vi "STAGE+mono+counter_edit26.vi"() -> ()   [LabVIEW 2017]
panel:
  out "Timeout":bool
  out "PROGRESS":u8(slide) max=10 step=10 scale=0.0..1.0
  in  "?":enum32{"Scan Data", "Scans", "RT Data"}(tab)
  out "Spectrum":cluster{dbl[], dbl[]}(graph)
  out "Decay":cluster{dbl[], dbl[]}[](graph)
  in  "Collect Data!":bool
  out "Waveform Graph":waveform(dbl)[](graph)
  out "?":i32(knob) scale=0.0..1000000.0
  out "Photon Counts":dbl
  in  "Wavelength":dbl
  in  "Show Real Time Data":bool
  in  "?":enum32{"DELAY", "COUNTER", "MONO", "PLOT"}(tab)
  in  "Data File Path":path
  out "Final time [ps]":dbl
  out "Current time [ps]":dbl
  out "Initial time [ps]":dbl
  in  "Set this as t0":bool
  in  "Axis":i32=1
  in  "Motor ON":bool
  in  "Motor OFF":bool
  out "Current Position [mm]":dbl
  out "Final Position [mm]":dbl
  in  "Data Points":i32=100
  out "Current Point":i32
  in  "Step Size [um]":i32=10
  in  "Target [mm]":dbl format="%.3f"
  in  "Move":bool
  out "Initial position [mm]":dbl
  in  "GPIB address":string="23"
  in  "Count Mode":u16(ring) items=["A,B for Preset T", "A-B for Preset T", "A+B for Preset T", "A for Preset B"]
  in  "Trigger mode":u16(ring) items=["10 MHz"=0, "Input 2"=2, "Input T"=3]
  in  "Channel A Input":u16(ring)=1 items=["10 MHz", "Input 1"]
  in  "Channel B Input":u16(ring)=2 items=["Input 1"=1, "Input 2"=2]
  in  "Number of Measurements\n to take at one point/ Number of Periods":u16=1 min=1 max=2000 step=1
  in  "Time between measurements\n at one point (s)/Dwell Time":dbl=0.002 min=0.002 max=60.0 step=0.001
  in  "gate mode (CW:0)":i16(slide) scale=0.0..2.0 scale format="%.2f"
  out "Counts":i32
  in  "Integrating time \nin 10^-7 sec":dbl=10000000.0
  in  "Discriminator Level (mV)":dbl min=-300.0 max=300.0 step=0.2
  in  "Discriminator Slope":bool
  in  "Channel":i16 min=0 max=2 step=1
  out "Grating #":dbl
  out "Blaze angle":dbl
  out "Grooves/mm":dbl
  out "Mono port":T1(ring)
  out "Time delay":u32=450000 min=1
  in  "Step size":dbl=10.0 min=0.0
  in  "Scan to":i32=4000
  in  "Scan from":i32=2600
  out "Current wavelength":dbl
  in  "?":bool
  in  "NEW UNIT":T2(ring)
  in  "Array":dbl[](array[numeric])
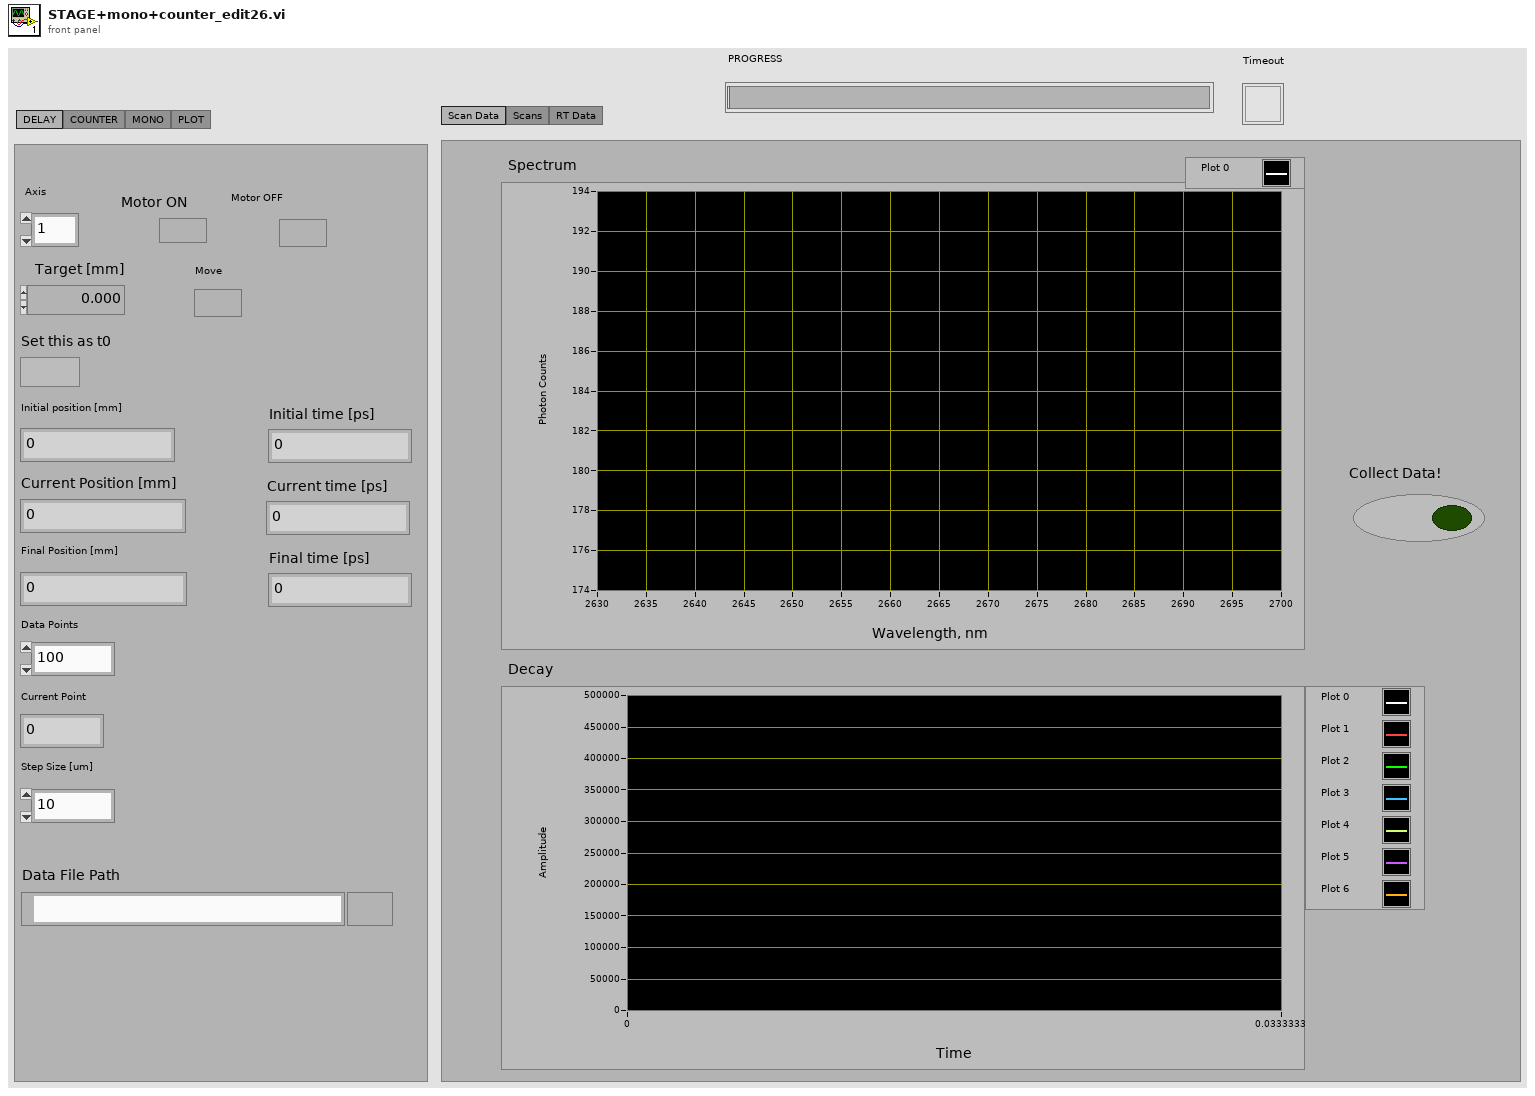
[diagram p1: front panel]
types:
  T1 = enum8{"COM 1", "COM 2", "COM 3", "COM 4", "COM 5", "COM 6", "COM 7", "COM 8", "COM 9"}
  T2 = enum16{"centi-Microns", " Nanometers", "   Angstroms"}
  T3 = cluster{"input XON/XOFF":bool, "input HW Handshake":bool, "input alt HW HShk":bool, "output XON/XOFF":bool, "output HW Handshake":bool, "output alt HW HShk":bool, "XOFF byte":u8, "XON byte":u8, "parity error byte":u16}
  T4 = enum16{"no parity", "odd parity", "even parity", "mark parity", "space parity"}
  T5 = enum16{"open", "replace", "create", "open or create", "replace or create", "replace or create with confirmation"}
  T6 = typedef "NI_Matrix.lvlib/RealMatrix.ctl" = dbl[][]
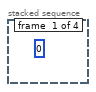
[diagram p2: hidden frame]
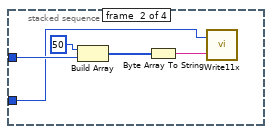
[diagram p3: hidden frame]
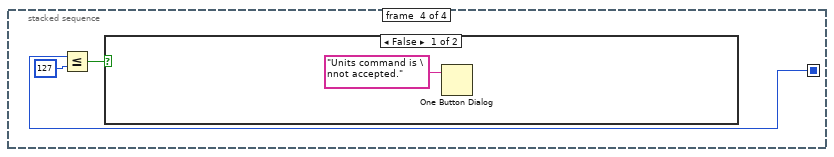
[diagram p4: hidden frame]
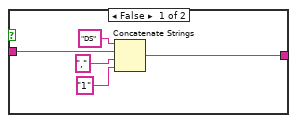
[diagram p7: hidden frame]
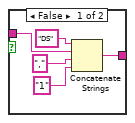
[diagram p9: hidden frame]
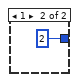
[diagram p13: hidden frame]
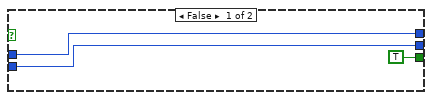
[diagram p14: hidden frame]
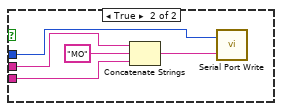
[diagram p15: hidden frame]
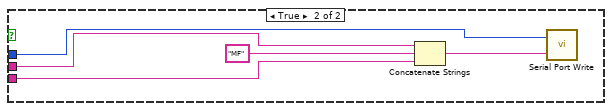
[diagram p16: hidden frame]
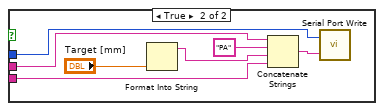
[diagram p17: hidden frame]
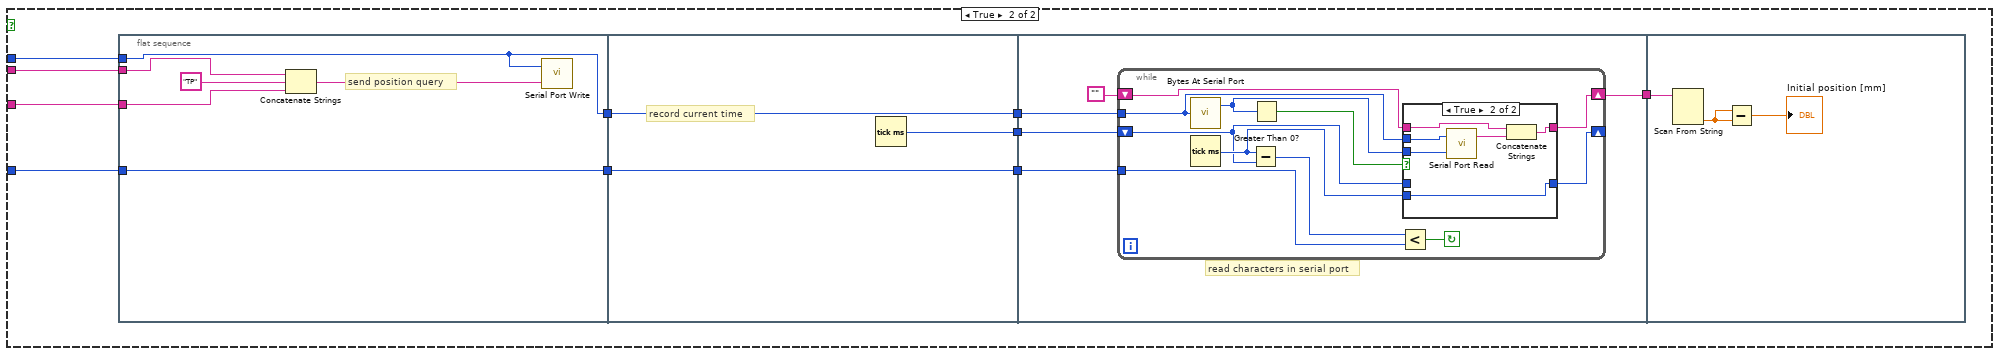
[diagram p18: hidden frame]
diagram:
  w35 = u32 19200  # baud rate
  w34 = u16 8  # data bits
  w33 = enum16{"1 bit", "1.5 bits", "2 bits"}."1 bit"  # stop bits
  w37 = T4."no parity"  # parity
  w17 = 4  # 0=COM1 so n=COM(n+1)
  w36 = u16 1024  # buffer size
  n1 = flat-sequence {
    tunnel: [w40] -> w9
    tunnel: [w39] -> w10
    frame #0 {
      n2 = call "CM Com Read ini.vi"() -> ("Mono port"=w39:T1, "time delay1"=w40:u32)  [unwired: 7 in]
    }
  }
  n3 = stacked-sequence {
    seq-local: [_ _ w48 _] -> [_ _ _ w55]
    tunnel: "NEW UNIT" -> [_ w42 _ _]
    tunnel: w9 -> [_ w41 w46 _]
    tunnel: w10 -> [_ _ w47 _]
    frame #0 {
      (unwired) u8 0
    }
    frame #1 {
      n4 = Build Array(u8 50, w42) -> (w44:u16[])
      n5 = Byte Array To String(unsigned byte array=w44) -> (string=w43:string)
      n6 = call "Write11x.vi"("string to write"=w43, "port number"=w41) -> ()  [unwired: 1 out]
    }
    frame #2 {
      n7 = call "Read11x.vi"("response size"=2, "timeout count"=w47, "port number"=w46) -> ("rcv index"=w49:u8[])  [unwired: 2 out]
      n8 = Index Array(array=w49, index=1) -> ()  [unwired: 1 out]
      n9 = Index Array(array=w49, index=0) -> (element=w48:u8)
    }
    frame #3 {
      n10 = Less Or Equal?(x=w55, y=127) -> (x <= y?=w53:bool)
      n11 = case shown="False" w53 {
        frame False {
          n12 = One Button Dialog(message="Units command is \nnot accepted.") -> ()  [unwired: 1 in, 1 out]
        }
        frame True {
        }
      }
    }
  }
  n13 = call "CM Serial Port Setup.vi"("COM port"=w10, "time delay"=w9) -> ("time delay1"=w1:u32, "DK port Out"=w2:T1, "error code"=w28:i32)  [unwired: 7 in]
  n14 = Equal To 0?(x=w28) -> (x = 0?=w27:bool)
  n15 = case shown="True" w27 {
    tunnel: w2 -> [w59 w62]
    tunnel: w1 -> [w58 w61]
    tunnel: [w59 w62] -> w14
    tunnel: [w58 w61] -> w13
    tunnel: [TRUE FALSE] -> w12
    frame False {
    }
    frame True {
      n16 = call "CM Com Write ini.vi"("time delay1"=w62, "Mono port"=w61) -> ()  [unwired: 7 in]
      n17 = local write "Mono port"(w62) -> ()
      n18 = local write "Time delay"(w61) -> ()
    }
  }
  n19 = call "Query11x.vi"("port number"=w2, "QUERY"=u16 4, "time delay"=w1) -> ("STATUS MESSAGE"=→"Grating #":u16)  [unwired: 3 out]
  n20 = call "Query11x.vi"("port number"=w2, "QUERY"=u16 2, "time delay"=w1) -> ("STATUS MESSAGE"=→"Grooves/mm":u16)  [unwired: 3 out]
  n21 = call "Query11x.vi"("port number"=w2, "QUERY"=u16 3, "time delay"=w1) -> ("STATUS MESSAGE"=→"Blaze angle":u16)  [unwired: 3 out]
  n22 = call <vilib>:"Serial Port Init.vi"("flow control etc."=T3 {"input XON/XOFF"=FALSE, "input HW Handshake"=FALSE, "input alt HW HShk"=FALSE, "output XON/XOFF"=FALSE, "output HW Handshake"=FALSE, "output alt HW HShk"=FALSE, "XOFF byte"=13, "XON byte"=11, "parity error byte"=0}, "parity"=w37, "buffer size"=w36, "stop bits"=w33, "data bits"=w34, "baud rate"=w35, "port number"=w17) -> ("error code"=w32:i32)
  n23 = Concatenate Strings("\r", "\n") -> (w29:string)
  n24 = while {
    tunnel: w13 -> [w65]
    tunnel: w14 -> [w64]
    stop <- TRUE continue-if-true
    n25 = case shown="True" "?" {
      tunnel: w65 -> [_ w68]
      tunnel: w64 -> [_ w67]
      frame False {
      }
      frame True {
        n26 = Two Button Dialog(message="Do you want to change grating?", 1:"No" ("F button name (\"Cancel\")"), 2:"Yes" ("T button name (\"OK\")")) -> (T button?=w69:bool)
        n27 = case shown="True" w69 {
          tunnel: w68 -> [_ w74]
          tunnel: w67 -> [_ w73]
          frame False {
          }
          frame True {
            n28 = Two Button Dialog(message="Disable voltage from PMT", 1:"Do not swich grating" ("F button name (\"Cancel\")"), 2:"Done" ("T button name (\"OK\")")) -> (T button?=w75:bool)
            n29 = case shown="True" w75 {
              tunnel: w74 -> [_ w87]
              tunnel: w73 -> [_ w86]
              frame False {
              }
              frame True {
                n30 = flat-sequence {
                  tunnel: w87 -> [w91]
                  tunnel: [w91] -> w81
                  tunnel: w86 -> [w90]
                  tunnel: [w90] -> w80
                  tunnel: [w88] -> w79
                  tunnel: w81 -> [w96]
                  tunnel: [w96] -> w84
                  tunnel: w80 -> [w97]
                  tunnel: [w97] -> w83
                  tunnel: w79 -> [w95]
                  tunnel: [w95] -> w82
                  tunnel: w84 -> [w101]
                  tunnel: w83 -> [w102]
                  tunnel: [w100] -> w85
                  tunnel: w82 -> [w100]
                  frame #0 {
                    n31 = local read "Grating #"() -> (w89:dbl)
                    n32 = case shown="2, Default" w89 {
                      tunnel: [1 2] -> w88
                      frame 2, Default {
                      }
                      frame 1 {
                      }
                    }
                    n33 = call "Select11x2.vi"("time delay"=w91, "NEW GRT?"=w88, "port number"=w90) -> ()  [unwired: 3 out]
                  }
                  frame #1 {
                    n34 = call "Query11x.vi"("port number"=w97, "QUERY"=u16 2, "time delay"=w96) -> ("STATUS MESSAGE"=w94:u16)  [unwired: 3 out]
                    n35 = local write "Grooves/mm"(w94) -> ()
                  }
                  frame #2 {
                    n36 = Divide(x=w101, y=i16 100 ("device (1)")) -> (x/y=w103:dbl)
                    n37 = call "Query11x.vi"("port number"=w102, "QUERY"=u16 3, "time delay"=w103) -> ("STATUS MESSAGE"=w99:u16)  [unwired: 3 out]
                    n38 = local write "Blaze angle"(w99) -> ()
                  }
                }
                n39 = local write "Grating #"(w85) -> ()
              }
            }
          }
        }
      }
    }
  }
  n40 = while {
    tunnel: w17 -> [w120]
    tunnel: w29 -> [w121]
    tunnel: w32 -> [_]
    tunnel: "Axis" -> [w118]
    stop <- TRUE continue-if-true
    w119 = u32 200  # timeout
    n41 = Format Into String(w118) -> (resulting string=w122:string)  [unwired: 3 in, 1 out]
    n42 = flat-sequence {
      tunnel: w122 -> [w127]
      tunnel: w121 -> [w126]
      tunnel: w120 -> [w128]
      tunnel: w119 -> [w125]
      tunnel: [w127] -> w117
      tunnel: [w126] -> w116
      tunnel: [w128] -> w115
      tunnel: [w125] -> w114
      tunnel: w117 -> [w138]
      tunnel: w116 -> [w137]
      tunnel: w115 -> [w139]
      tunnel: w114 -> [w135]
      tunnel: [w138] -> w113
      tunnel: [w137] -> w112
      tunnel: [w139] -> w111
      tunnel: [w135] -> w110
      tunnel: w113 -> [w148]
      tunnel: w112 -> [w147]
      tunnel: w111 -> [w149]
      tunnel: w110 -> [w145]
      tunnel: [w148] -> w109
      tunnel: [w147] -> w108
      tunnel: [w149] -> w107
      tunnel: [w145] -> w106
      tunnel: w109 -> [w161]
      tunnel: w108 -> [w158]
      tunnel: w107 -> [w160]
      tunnel: w106 -> [w159]
      frame #0 {
        n43 = case shown="False" "Motor ON" {
          tunnel: w128 -> [_ w134]
          tunnel: w127 -> [_ w131]
          tunnel: w126 -> [_ w130]
          frame False {
          }
          frame True {
            n44 = Concatenate Strings(w131, "MO" ("Substring"), w130) -> (w132:string)
            n45 = call <vilib>:"Serial Port Write.vi"("string to write"=w132, "port number"=w134) -> ()  [unwired: 1 out]
          }
        }
      }
      frame #1 {
        n46 = case shown="False" "Motor OFF" {
          tunnel: w139 -> [_ w144]
          tunnel: w138 -> [_ w141]
          tunnel: w137 -> [_ w140]
          frame False {
          }
          frame True {
            n47 = Concatenate Strings(w141, "MF" ("Substring"), w140) -> (w142:string)
            n48 = call <vilib>:"Serial Port Write.vi"("string to write"=w142, "port number"=w144) -> ()  [unwired: 1 out]
          }
        }
      }
      frame #2 {
        n49 = case shown="False" "Move" {
          tunnel: w149 -> [_ w156]
          tunnel: w148 -> [_ w153]
          tunnel: w147 -> [_ w152]
          frame False {
          }
          frame True {
            n50 = Format Into String("Target [mm]") -> (resulting string=w150:string)  [unwired: 3 in, 1 out]
            n51 = Concatenate Strings(w153, "PA" ("Substring"), w150, w152) -> (w154:string)
            n52 = call <vilib>:"Serial Port Write.vi"("string to write"=w154, "port number"=w156) -> ()  [unwired: 1 out]
          }
        }
      }
      frame #3 {
        n53 = case shown="False" "Set this as t0" {
          tunnel: w161 -> [_ w171]
          tunnel: w160 -> [_ w170]
          tunnel: w159 -> [_ w169]
          tunnel: w158 -> [_ w168]
          frame False {
          }
          frame True {
            n54 = flat-sequence {
              tunnel: w171 -> [w175]
              tunnel: w170 -> [w174]
              tunnel: [w174] -> w167
              tunnel: w169 -> [w172]
              tunnel: [w172] -> w166
              tunnel: w168 -> [w173]
              tunnel: w167 -> [w179]
              tunnel: [w179] -> w165
              tunnel: w166 -> [w178]
              tunnel: [w178] -> w164
              tunnel: [w180] -> w163
              tunnel: w165 -> [w185]
              tunnel: w164 -> [w183]
              tunnel: w163 -> [w182]
              tunnel: [w181] -> w162
              tunnel: w162 -> [w207]
              frame #0 {
                # "send position query"
                n55 = Concatenate Strings(w175, "TP" ("Substring"), w173) -> (w176:string)
                n56 = call <vilib>:"Serial Port Write.vi"("string to write"=w176, "port number"=w174) -> ()  [unwired: 1 out]
              }
              frame #1 {
                # "record current time"
                n57 = Tick Count (ms)() -> (millisecond timer value=w180:u32)
              }
              frame #2 {
                # "read characters in serial port"
                n58 = while {
                  shift-left: w182 -> [w186]
                  shift-right: [w187] -> _
                  tunnel: w183 -> [w190]
                  shift-left: "" -> [w193]
                  shift-right: [w192] -> w181
                  tunnel: w185 -> [w194]
                  stop <- w189 continue-if-true
                  n59 = call <vilib>:"Bytes At Serial Port.vi"("port number"=w194) -> ("byte count"=w195:u32)  [unwired: 1 out]
                  n60 = Tick Count (ms)() -> (millisecond timer value=w188:u32)
                  n61 = Subtract(x=w188, y=w186) -> (x-y=w191:u32)
                  n62 = Greater Than 0?(x=w195) -> (x > 0?=w196:bool)
                  n63 = Less?(x=w191, y=w190) -> (x < y?=w189:bool)
                  n64 = case shown="True" w196 {
                    tunnel: w195 -> [_ w204]
                    tunnel: w194 -> [_ w203]
                    tunnel: w193 -> [w198 w201]
                    tunnel: [w198 w200] -> w192
                    tunnel: [w197 w199] -> w187
                    tunnel: w188 -> [_ w199]
                    tunnel: w186 -> [w197 _]
                    frame False {
                    }
                    frame True {
                      n65 = call <vilib>:"Serial Port Read.vi"("requested byte count"=w204, "port number"=w203) -> ("string read"=w202:string)  [unwired: 1 out]
                      n66 = Concatenate Strings(w201, w202) -> (w200:string)
                    }
                  }
                }
              }
              frame #3 {
                n67 = Scan From String(input string=w207) -> (output 1=w205:dbl)  [unwired: 4 in, 3 out]
                n68 = Subtract(x=w205, y=w205) -> (x-y=→"Initial position [mm]":dbl)
              }
            }
          }
        }
      }
    }
    n69 = Wait Until Next ms Multiple(millisecond multiple=u32 50) -> ()  [unwired: 1 out]
  }
  n70 = while {
    tunnel: "GPIB address" -> [w211]
    tunnel: w14 -> [w210]
    tunnel: w13 -> [w209]
    tunnel: w12 -> [w208]
    stop <- TRUE continue-if-true
    n71 = case shown="True" "Show Real Time Data" {
      tunnel: w211 -> [_ w220]
      tunnel: w210 -> [_ w217]
      tunnel: w209 -> [_ w214]
      tunnel: w208 -> [_ w219]
      frame False {
      }
      frame True {
        n72 = flat-sequence {
          tunnel: w220 -> [w249]
          tunnel: "Wavelength" -> [w250]
          tunnel: [w250] -> w231
          tunnel: [w239] -> w230
          tunnel: [w240] -> w229
          tunnel: [w249] -> w228
          tunnel: w214 -> [w240]
          tunnel: w217 -> [w239]
          tunnel: w219 -> [_]
          tunnel: [w238] -> w215
          tunnel: w214 -> [w238]
          tunnel: [w258] -> w227
          tunnel: [w257] -> w226
          tunnel: [w255] -> w225
          tunnel: w231 -> [w253]
          tunnel: w230 -> [w258]
          tunnel: w229 -> [w257]
          tunnel: w228 -> [w255]
          tunnel: [w251] -> w216
          tunnel: w215 -> [w251]
          tunnel: w227 -> [_]
          tunnel: w226 -> [_]
          tunnel: w225 -> [w261]
          tunnel: [w261] -> w224
          tunnel: w217 -> [w260]
          tunnel: w216 -> [w259]
          tunnel: w224 -> [w270]
          tunnel: [w270] -> w223
          tunnel: w223 -> [w320]
          tunnel: [w320] -> w222
          tunnel: w222 -> [w321]
          tunnel: [w321] -> w221
          tunnel: w221 -> [w331]
          frame #0 {
            n73 = call "Query11x.vi"("port number"=w239, "QUERY"=u16 0, "time delay"=w240) -> ("timeout"=w236:bool, "STATUS MESSAGE"=w235:u16)  [unwired: 2 out]
            n74 = call "Query11x.vi"("port number"=w239, "QUERY"=u16 2, "time delay"=w240) -> ("timeout"=w247:bool, "STATUS MESSAGE"=w246:u16)  [unwired: 2 out]
            n75 = call "Query11x.vi"("port number"=w239, "QUERY"=u16 4, "time delay"=w240) -> ("timeout"=w241:bool, "STATUS MESSAGE"=w242:u16)  [unwired: 2 out]
            n76 = call "Query11x.vi"("port number"=w239, "QUERY"=u16 3, "time delay"=w240) -> ("timeout"=→"Timeout":bool, "STATUS MESSAGE"=w244:u16)  [unwired: 2 out]
            n77 = local write "Timeout"(w236) -> ()
            n78 = local write "Timeout"(w247) -> ()
            n79 = local write "Grooves/mm"(w246) -> ()
            n80 = local write "Timeout"(w241) -> ()
            n81 = local write "Grating #"(w242) -> ()
            n82 = Divide(x=w235, y=10 ("Numeric")) -> (x/y=w233:dbl)
            n83 = local write "Current wavelength"(w233) -> ()
            n84 = local write "Blaze angle"(w244) -> ()
          }
          frame #1 {
            n85 = Multiply(x=w253, y=1) -> (x*y=w252:dbl)
            n86 = call "Goto11x.vi"("time delay"=w257, "WAVELENGTH"=w252, "port number"=w258) -> ("timeout"=w256:bool)  [unwired: 2 out]
            n87 = local write "Timeout"(w256) -> ()
          }
          frame #2 {
            # "set counter time in 10^-7 seconds in CW"
            n88 = call "Query11x.vi"("port number"=w260, "QUERY"=0, "time delay"=w259) -> ("timeout"=w265:bool, "STATUS MESSAGE"=w264:u16)  [unwired: 2 out]
            n89 = local write "Timeout"(w265) -> ()
            n90 = Divide(x=w264, y=1) -> (x/y=w263:dbl)
            n91 = local write "Current wavelength"(w263) -> ()
          }
          frame #3 {
            # "Configures discriminator."
            n92 = flat-sequence {
              tunnel: w270 -> [w277]
              tunnel: [w277] -> w276
              tunnel: [w284] -> w275
              tunnel: [w282] -> w274
              tunnel: w269 -> [w283]
              tunnel: w276 -> [w282]
              tunnel: w271 -> [w281]
              tunnel: w275 -> [w303]
              tunnel: [w304] -> w273
              tunnel: w274 -> [w302]
              tunnel: [w302] -> w272
              tunnel: w271 -> [w300]
              tunnel: w273 -> [w316]
              tunnel: w272 -> [w315]
              tunnel: w267 -> [w310]
              tunnel: w271 -> [w309]
              frame #0 {
                # "Flush I/O buffers."
                n93 = for {
                  N: 5 -> [_]
                  tunnel: w277 -> [w279]
                  n94 = GPIB Write(0:w279, 1:"\r") -> ()  [unwired: 3 in, 2 out]
                }
              }
              frame #1 {
                # "Set discriminator slope."
                n95 = case shown="True" w283 {
                  tunnel: [w290 w295] -> w285
                  tunnel: w281 -> [w289 w294]
                  frame False {
                    n96 = Concatenate Strings("DS", w289, ",", "1") -> (w290:string)
                  }
                  frame True {
                    n97 = Concatenate Strings("DS", w294, ",", "0") -> (w295:string)
                  }
                }
                n98 = GPIB Write(0:w282, 1:w285, 2:5) -> (6:w284:errorcluster)  [unwired: 2 in, 1 out]
              }
              frame #2 {
                # "Set discriminator mode to fixed."
                n99 = Concatenate Strings("DM", w300, ",", "0") -> (w299:string)
                n100 = GPIB Write(0:w302, 1:w299, 2:5, 3:w303) -> (6:w304:errorcluster)  [unwired: 1 in, 1 out]
              }
              frame #3 {
                # "Set discriminator level.\nMust be between +300 and -300 mV."
                n101 = Divide(x=w310, y=1000.0) -> (x/y=w318:dbl)
                n102 = Number To Fractional String(number=w318, precision (6)=i16 4) -> (F-format string=w307:string)  [unwired: 2 in]
                n103 = Concatenate Strings("DL", w309, ",", w307) -> (w314:string)
                n104 = GPIB Write(0:w315, 1:w314, 2:5, 3:w316) -> (6:w311:errorcluster)  [unwired: 1 in, 1 out]
                n105 = call <vilib>:"General Error Handler.vi"("type of dialog (OK msg:1)"=1, "error in (no error)"=w311) -> ()  [unwired: 9 in, 5 out]
              }
            }
            n106 = local read "Discriminator Slope"() -> (w269:bool)
            n107 = local read "Channel"() -> (w268:i16)
            n108 = Number To Decimal String(number=w268) -> (decimal integer string=w271:string)  [unwired: 1 in]
            n109 = local read "Discriminator Level (mV)"() -> (w267:dbl)
          }
          frame #4 {
            n110 = call "Start.vi"("GPIB Address"=w320) -> ()  [unwired: 9 in]
          }
          frame #5 {
            # "Wait for Scan to Finish"
            n111 = for {
              N: 1 -> [_]
              tunnel: w321 -> [w323]
              n112 = while {
                tunnel: w323 -> [w324]
                stop <- w326 stop-if-true
                n113 = call "ScanDone.vi"("Wait (ms)"=1000, "GPIB Address"=w324) -> ("Scan Finished?"=w326:bool)
              }
            }
          }
          frame #6 {
            n114 = call "Read Data.vi"("Channel Number"=0, "GPIB Address"=w331, "Number of Datapoints"=1) -> ("Data"=w332:i32[])
            n115 = property class="Knob (strict)"("Scale.Increment"=1000, "Scale.Maximum"=1000000, "Scale.Minimum"=0) -> ()  [unwired: 2 in, 2 out]
            n116 = Index Array(array=w332, index=0) -> (element=→"Photon Counts" →"?":i32)
          }
        }
      }
    }
  }
  n117 = while {
    tunnel: "Axis" -> [w344]
    tunnel: w17 -> [w343]
    tunnel: "GPIB address" -> [w342]
    tunnel: "Integrating time \nin 10^-7 sec" -> [w341]
    tunnel: w13 -> [w340]
    tunnel: w14 -> [w339]
    tunnel: w12 -> [w338]
    stop <- TRUE continue-if-true
    n118 = case shown="True" "Collect Data!" {
      selector: "Collect Data!" -> [_ w345]
      tunnel: w344 -> [_ w353]
      tunnel: w343 -> [_ w352]
      tunnel: w342 -> [_ w351]
      tunnel: w342 -> [_ w349]
      tunnel: w341 -> [_ w348]
      tunnel: w340 -> [_ w347]
      tunnel: w339 -> [_ w350]
      tunnel: w338 -> [_ w346]
      frame False {
      }
      frame True {
        n119 = flat-sequence {
          tunnel: w353 -> [w373]
          tunnel: w352 -> [w371]
          tunnel: w351 -> [w370]
          tunnel: w350 -> [w369]
          tunnel: w349 -> [w368]
          tunnel: w348 -> [w365]
          tunnel: w347 -> [w358]
          tunnel: w346 -> [w357]
          tunnel: w345 -> [_]
          frame #0 {
            w378 = 1000000000000.0
            w383 = 1000
            w384 = 300000000
            w390 = 1
            n120 = Multiply(x="Step Size [um]", y="Data Points") -> (x*y=w387:i32)
            n121 = Divide(x="Step Size [um]", y=1000.0) -> (x/y=w396:dbl)
            n122 = local read "Initial position [mm]"() -> (w375:dbl)
            n123 = Multiply(x="Scan to", y=w390) -> (x*y=w364:i32)
            n124 = Increment(x="Data Points") -> (x+1=w405:i32)
            n125 = Multiply(x="Scan from", y=w390) -> (x*y=w363:i32)
            n126 = Divide(x=w387, y=1000) -> (x/y=w386:dbl)
            n127 = To Time Stamp(1:w363) -> (0:w393:timestamp)
            n128 = Multiply(x=w364, y=1) -> (x*y=w402:i32)
            n129 = Multiply(x=1, y=w363) -> (x*y=w367:i32)
            n130 = Divide(x=w396, y=1000.0) -> (x/y=w397:dbl)
            n131 = for {
              N: w405 -> [_]
              tunnel: w396 -> [w761]
              tunnel: w375 -> [w759]
              tunnel: [w752] -> w404 mode=indexing
              i -> [w760]
              # "distances"
              n132 = Multiply(x=w761, y=w760) -> (x*y=w758:dbl)
              n133 = Add(x=w759, y=w758) -> (x+y=w757:dbl)
              n134 = Divide(x=w757, y=1000) -> (x/y=w751:dbl)
              n135 = Divide(x=w751, y=300000000) -> (x/y=w754:dbl)
              n136 = Multiply(x=w754, y=1000000000000.0) -> (x*y=w752:dbl)
            }
            n137 = Subtract(x=w402, y=w367) -> (x-y=w408:i32)
            n138 = Divide(x=w375, y=w383) -> (x/y=w381:dbl)
            n139 = Add(x=w375, y=w386) -> (x+y=w377:dbl)
            "Final Position [mm]" <- w377
            n140 = property on="Waveform Graph" class="WFGraph (strict)"("XScale.Increment"="Step size", "XScale.Maximum"=w364, "XScale.Minimum"=w363) -> ()  [unwired: 2 in, 2 out]
            n141 = Divide(x=w377, y=w383) -> (x/y=w382:dbl)
            n142 = Divide(x=w408, y="Step size") -> (x/y=w407:dbl)
            n143 = Divide(x=w381, y=w384) -> (x/y=w380:dbl)
            n144 = Divide(x=w397, y=300000000) -> (x/y=w399:dbl)
            n145 = Bundle By Name("Y"=dbl[] [], "t0"=w393, "dt"="Step size") -> (w392:waveform(dbl))  [unwired: 1 in]
            n146 = Divide(x=w382, y=w384) -> (x/y=w379:dbl)
            n147 = Multiply(x=w399, y=1000000000000.0) -> (x*y=w361:dbl)
            n148 = Multiply(x=w380, y=w378) -> (x*y=w360:dbl)
            "Initial time [ps]" <- w360
            n149 = Build Array(w392) -> (w356:waveform(dbl)[])
            n150 = Round Toward -Infinity(1:w407) -> (0:w366:dbl)
            n151 = Concatenate Strings("\r", "\n") -> (w372:string)
            n152 = Multiply(x=w379, y=w378) -> (x*y=w391:dbl)
            "Final time [ps]" <- w391
            n153 = Increment(x=w366) -> (x+1=w395:dbl)
            n154 = for {
              N: w395 -> [_]
              tunnel: "Step size" -> [w766]
              tunnel: w367 -> [w764]
              tunnel: [w762] -> _ mode=indexing
              i -> [w765]
              # "wavelengths"
              n155 = Multiply(x=w766, y=w765) -> (x*y=w763:dbl)
              n156 = Add(x=w764, y=w763) -> (x+y=w762:dbl)
            }
            n157 = for {
              N: "Data Points" -> [w432]
              tunnel: w375 -> [w473]
              tunnel: "Step Size [um]" -> [w469]
              tunnel: w373 -> [w466]
              tunnel: w372 -> [w463]
              tunnel: w371 -> [w464]
              tunnel: w370 -> [w462]
              tunnel: w369 -> [w460]
              tunnel: w368 -> [w461]
              tunnel: w367 -> [w423]
              tunnel: "Step size" -> [w455]
              tunnel: w366 -> [w454]
              tunnel: w365 -> [w453]
              tunnel: w364 -> [w418]
              tunnel: w363 -> [w417]
              tunnel: "Step size" -> [w419]
              tunnel: w361 -> [w434]
              tunnel: w360 -> [w451]
              shift-right: [w433] -> _
              shift-left: dbl[] [] -> [w429]
              tunnel: w358 -> [w446]
              tunnel: w369 -> [w445]
              tunnel: w357 -> [w444]
              shift-right: [w439] -> _
              shift-left: w356 -> [w440]
              shift-right: [w427] -> _
              shift-left: dbl[][] [] -> [w426]
              shift-right: [w415] -> _
              shift-left: dbl[][] [] -> [w413]
              i -> [w421]
              w443 = dbl[] []
              n158 = stacked-sequence {
                tunnel: w460 -> [w734]
                tunnel: w461 -> [_]
                frame #0 {
                  n159 = call <vilib>:"Close Serial Driver.vi"("port number"=w734) -> ()  [unwired: 1 out]
                  n160 = GPIB Misc(0:"loc 23" ("command string")) -> ()  [unwired: 1 in, 3 out]
                }
              }
              n161 = property on="Waveform Graph" class="WFGraph (strict)"("XScale.Increment"=w419, "XScale.Maximum"=w418, "XScale.Minimum"=w417) -> ()  [unwired: 2 in, 2 out]
              n162 = Number To Decimal String(number=w453) -> (decimal integer string=w458:string)  [unwired: 1 in]
              n163 = Divide(x=w469, y=1000) -> (x/y=w468:dbl)
              n164 = property on="PROGRESS" class="Slide (strict)"("Scale.Increment"=1, "Scale.Maximum"=w432, "Scale.Minimum"=0) -> ()  [unwired: 2 in, 2 out]
              n165 = Multiply(x=w434, y=w421) -> (x*y=w452:dbl)
              n166 = Add(x=1, y=w421) -> (x+y=→"PROGRESS":i32)
              n167 = Concatenate Strings("CP 2,", w458) -> (w456:string)
              n168 = Add(x=w451, y=w452) -> (x+y=w430:dbl)
              n169 = Multiply(x=w468, y=w421) -> (x*y=w472:dbl)
              n170 = Add(x=w473, y=w472) -> (x+y=w471:dbl)
              n171 = Build Array (concatenate)(w429, w430) -> (w431:dbl[])
              n172 = Format Into String(w466) -> (resulting string=w465:string)  [unwired: 3 in, 1 out]
              n173 = GPIB Write(0:w462, 1:w456, 2:i16 5 ("mode (0)")) -> ()  [unwired: 2 in, 2 out]
              n174 = flat-sequence {
                tunnel: w471 -> [w737]
                tunnel: [w737] -> w467
                tunnel: w463 -> [w739]
                tunnel: w465 -> [w738]
                tunnel: w464 -> [w735]
                tunnel: w467 -> [w748]
                tunnel: [w743] -> w416
                frame #0 {
                  n175 = Format Into String(w737) -> (resulting string=w736:string)  [unwired: 3 in, 1 out]
                  n176 = Wait (ms)(milliseconds to wait=u32 100) -> ()  [unwired: 1 out]
                  n177 = Concatenate Strings(w738, "PA" ("Substring"), w736, w739) -> (w741:string)
                  n178 = call <vilib>:"Serial Port Write.vi"("string to write"=w741, "port number"=w735) -> ()  [unwired: 1 out]
                }
                frame #1 {
                  n179 = Divide(x=w748, y=1000) -> (x/y=w746:dbl)
                  n180 = Wait (ms)(milliseconds to wait=u32 1000) -> ()  [unwired: 1 out]
                  n181 = Divide(x=w746, y=300000000) -> (x/y=w745:dbl)
                  n182 = Multiply(x=w745, y=1000000000000.0) -> (x*y=w743:dbl)
                  "Current time [ps]" <- w743
                  "Current Position [mm]" <- w748
                }
              }
              n183 = Add(x=w421, y=1) -> (x+y=w420:i32)
              n184 = flat-sequence {
                tunnel: w462 -> [w499]
                tunnel: w423 -> [w498]
                tunnel: w455 -> [w497]
                tunnel: w454 -> [w496]
                tunnel: w418 -> [w495]
                tunnel: w417 -> [w494]
                tunnel: w443 -> [w493]
                tunnel: w443 -> [w492]
                tunnel: w419 -> [w491]
                tunnel: w446 -> [w490]
                tunnel: w445 -> [w489]
                tunnel: w444 -> [w488]
                tunnel: [w486] -> w442
                tunnel: [w487] -> _
                tunnel: [w486] -> w441
                tunnel: w420 -> [w485]
                tunnel: w416 -> [w484]
                tunnel: [w483] -> w414
                tunnel: w413 -> [w482]
                tunnel: w442 -> [w712]
                tunnel: [w715] -> w428
                tunnel: [w714] -> w425
                tunnel: [w713] -> w415
                tunnel: w414 -> [w713]
                frame #0 {
                  # "step size"
                  n185 = while {
                    tunnel: w499 -> [w541]
                    tunnel: w498 -> [w562]
                    tunnel: w497 -> [w534]
                    tunnel: w496 -> [w561]
                    tunnel: w495 -> [w537]
                    tunnel: w494 -> [w536]
                    tunnel: w491 -> [w538]
                    shift-right: [w558] -> w486
                    shift-left: w492 -> [w557]
                    shift-right: [w553] -> w487
                    shift-left: w493 -> [w560]
                    tunnel: w490 -> [w500]
                    tunnel: w489 -> [w501]
                    tunnel: w488 -> [w543]
                    tunnel: w485 -> [w522]
                    tunnel: w484 -> [w510]
                    shift-right: [w503] -> w483
                    shift-left: w482 -> [w502]
                    i -> [w530]
                    stop <- w532 stop-if-true
                    n186 = property on="Spectrum" class="XYGraph (strict)"("XScale.Increment"=w538, "XScale.Maximum"=w537, "XScale.Minimum"=w536) -> ()  [unwired: 2 in, 2 out]
                    n187 = Multiply(x=1, y=w534) -> (x*y=w533:dbl)
                    n188 = Multiply(x=w530, y=w533) -> (x*y=w563:dbl)
                    n189 = Greater Or Equal?(x=w530, y=w561) -> (x >= y?=w532:bool)
                    n190 = Add(x=w563, y=w562) -> (x+y=w542:dbl)
                    n191 = Add(x=w530, y=1) -> (x+y=w523:i32)
                    n192 = Build Array (concatenate)(w560, w542) -> (w559:dbl[])
                    n193 = flat-sequence {
                      tunnel: w541 -> [w574]
                      tunnel: w542 -> [w575]
                      tunnel: [w575] -> w547
                      tunnel: [w565] -> w546
                      tunnel: [w564] -> w545
                      tunnel: [w574] -> w544
                      tunnel: w500 -> [w564]
                      tunnel: w501 -> [w565]
                      tunnel: w543 -> [_]
                      tunnel: [w573] -> w524
                      tunnel: w523 -> [w573]
                      tunnel: [w572] -> w511
                      tunnel: w510 -> [w572]
                      tunnel: w502 -> [w571]
                      tunnel: [w571] -> w509
                      tunnel: [w585] -> w552
                      tunnel: [w584] -> w551
                      tunnel: [w582] -> w550
                      tunnel: w547 -> [w578]
                      tunnel: w546 -> [w585]
                      tunnel: w545 -> [w584]
                      tunnel: w544 -> [w582]
                      tunnel: [w579] -> w525
                      tunnel: w524 -> [w579]
                      tunnel: [w578] -> w517
                      tunnel: [w577] -> w512
                      tunnel: w511 -> [w577]
                      tunnel: w509 -> [w576]
                      tunnel: [w576] -> w508
                      tunnel: w552 -> [_]
                      tunnel: w551 -> [_]
                      tunnel: w550 -> [w592]
                      tunnel: [w592] -> w540
                      tunnel: [w591] -> w526
                      tunnel: w525 -> [w591]
                      tunnel: [w590] -> w518
                      tunnel: w517 -> [w590]
                      tunnel: [w589] -> w513
                      tunnel: w512 -> [w589]
                      tunnel: w508 -> [w588]
                      tunnel: [w588] -> w507
                      tunnel: w501 -> [w587]
                      tunnel: w500 -> [w586]
                      tunnel: w540 -> [w602]
                      tunnel: [w602] -> w539
                      tunnel: [w601] -> w527
                      tunnel: w526 -> [w601]
                      tunnel: [w600] -> w519
                      tunnel: w518 -> [w600]
                      tunnel: [w599] -> w514
                      tunnel: w513 -> [w599]
                      tunnel: w507 -> [w598]
                      tunnel: [w598] -> w506
                      tunnel: w539 -> [w659]
                      tunnel: [w659] -> w549
                      tunnel: [w658] -> w528
                      tunnel: w527 -> [w658]
                      tunnel: [w657] -> w520
                      tunnel: w519 -> [w657]
                      tunnel: [w656] -> w515
                      tunnel: w514 -> [w656]
                      tunnel: w506 -> [w655]
                      tunnel: [w655] -> w505
                      tunnel: w549 -> [w664]
                      tunnel: [w664] -> w548
                      tunnel: [w663] -> w529
                      tunnel: w528 -> [w663]
                      tunnel: [w662] -> w521
                      tunnel: w520 -> [w662]
                      tunnel: [w661] -> w516
                      tunnel: w515 -> [w661]
                      tunnel: w505 -> [w660]
                      tunnel: [w660] -> w504
                      tunnel: [w675] -> w555
                      tunnel: w548 -> [w707]
                      tunnel: w529 -> [w673]
                      tunnel: w522 -> [w676]
                      tunnel: w521 -> [w677]
                      tunnel: w516 -> [w679]
                      tunnel: w504 -> [w674]
                      tunnel: [w672] -> w503
                      frame #0 {
                        n194 = call "Query11x.vi"("port number"=w565, "QUERY"=u16 0, "time delay"=w564) -> ("timeout"=w569:bool, "STATUS MESSAGE"=w568:u16)  [unwired: 2 out]
                        n195 = local write "Timeout"(w569) -> ()
                        n196 = Divide(x=w568, y=1 ("Numeric")) -> (x/y=→"Current wavelength":dbl)
                      }
                      frame #1 {
                        n197 = Multiply(x=w578, y=1) -> (x*y=w580:dbl)
                        n198 = call "Goto11x.vi"("time delay"=w584, "WAVELENGTH"=w580, "port number"=w585) -> ("timeout"=w583:bool)  [unwired: 2 out]
                        n199 = local write "Timeout"(w583) -> ()
                      }
                      frame #2 {
                        # "set counter time in 10^-7 seconds in CW"
                        n200 = call "Query11x.vi"("port number"=w587, "QUERY"=0, "time delay"=w586) -> ("timeout"=w596:bool, "STATUS MESSAGE"=w595:u16)  [unwired: 2 out]
                        n201 = local write "Timeout"(w596) -> ()
                        n202 = Divide(x=w595, y=1) -> (x/y=w594:dbl)
                        n203 = local write "Current wavelength"(w594) -> ()
                      }
                      frame #3 {
                        # "Configures discriminator."
                        n204 = flat-sequence {
                          tunnel: w602 -> [w612]
                          tunnel: [w612] -> w611
                          tunnel: [w619] -> w610
                          tunnel: [w617] -> w609
                          tunnel: "Discriminator Slope" -> [w618]
                          tunnel: w611 -> [w617]
                          tunnel: w603 -> [w616]
                          tunnel: w610 -> [w638]
                          tunnel: [w639] -> w608
                          tunnel: w609 -> [w637]
                          tunnel: [w637] -> w607
                          tunnel: w603 -> [w635]
                          tunnel: w608 -> [w651]
                          tunnel: w607 -> [w650]
                          tunnel: "Discriminator Level (mV)" -> [w645]
                          tunnel: w603 -> [w644]
                          frame #0 {
                            # "Flush I/O buffers."
                            n205 = for {
                              N: 5 -> [_]
                              tunnel: w612 -> [w614]
                              n206 = GPIB Write(0:w614, 1:"\r") -> ()  [unwired: 3 in, 2 out]
                            }
                          }
                          frame #1 {
                            # "Set discriminator slope."
                            n207 = case shown="True" w618 {
                              tunnel: [w625 w630] -> w620
                              tunnel: w616 -> [w624 w629]
                              frame False {
                                n208 = Concatenate Strings("DS", w624, ",", "1") -> (w625:string)
                              }
                              frame True {
                                n209 = Concatenate Strings("DS", w629, ",", "0") -> (w630:string)
                              }
                            }
                            n210 = GPIB Write(0:w617, 1:w620, 2:5) -> (6:w619:errorcluster)  [unwired: 2 in, 1 out]
                          }
                          frame #2 {
                            # "Set discriminator mode to fixed."
                            n211 = Concatenate Strings("DM", w635, ",", "0") -> (w634:string)
                            n212 = GPIB Write(0:w637, 1:w634, 2:5, 3:w638) -> (6:w639:errorcluster)  [unwired: 1 in, 1 out]
                          }
                          frame #3 {
                            # "Set discriminator level.\nMust be between +300 and -300 mV."
                            n213 = Divide(x=w645, y=1000.0) -> (x/y=w653:dbl)
                            n214 = Number To Fractional String(number=w653, precision (6)=i16 4) -> (F-format string=w642:string)  [unwired: 2 in]
                            n215 = Concatenate Strings("DL", w644, ",", w642) -> (w649:string)
                            n216 = GPIB Write(0:w650, 1:w649, 2:5, 3:w651) -> (6:w646:errorcluster)  [unwired: 1 in, 1 out]
                            n217 = call <vilib>:"General Error Handler.vi"("type of dialog (OK msg:1)"=1, "error in (no error)"=w646) -> ()  [unwired: 9 in, 5 out]
                          }
                        }
                        n218 = Number To Decimal String(number="Channel") -> (decimal integer string=w603:string)  [unwired: 1 in]
                      }
                      frame #4 {
                        n219 = call "Start.vi"("GPIB Address"=w659) -> ()  [unwired: 9 in]
                      }
                      frame #5 {
                        # "Wait for Scan to Finish"
                        n220 = for {
                          N: 1 -> [_]
                          tunnel: w664 -> [w666]
                          n221 = while {
                            tunnel: w666 -> [w667]
                            stop <- w669 stop-if-true
                            n222 = call "ScanDone.vi"("Wait (ms)"=1000, "GPIB Address"=w667) -> ("Scan Finished?"=w669:bool)
                          }
                        }
                      }
                      frame #6 {
                        w678 = 0
                        w686 = "\r\n"
                        n223 = call "Read Data.vi"("Channel Number"=0, "GPIB Address"=w707, "Number of Datapoints"=1) -> ("Data"=w708:i32[])
                        n224 = Index Array(array=w708, index=0) -> (element=w675:i32)
                        "Counts" <- w675
                        n225 = local read "Integrating time \nin 10^-7 sec"() -> (w684:dbl)
                        n226 = Replace Array Subset(array=w674, new element #1=w675, index (row) #1=w673, index (col) #1=w676, new element #2=w677, index (row) #2=w673, index (col) #2=w678, new element #3=w679, index (row) #3=w678, index (col) #3=w676) -> (w672:T6)
                        n227 = Array To Spreadsheet String(delimiter (Tab)=",", array=w672, 3:"%f" ("format string")) -> (spreadsheet string=w685:string)
                        n228 = local read "Blaze angle"() -> (w702:dbl)
                        n229 = local read "Grating #"() -> (w701:dbl)
                        n230 = Multiply(x=w684, y=1e-07) -> (x*y=w683:dbl)
                        n231 = Get Date/Time In Seconds() -> (seconds since 1Jan1904=w696:timestamp)
                        n232 = Format Date/Time String(time format string (%c)="%Y-%b-%d %H:%M:%S", seconds (now)=w696) -> (date/time string=w697:string)  [unwired: 1 in]
                        n233 = Number To Decimal String(number=w683) -> (decimal integer string=w698:string)  [unwired: 1 in]
                        n234 = Number To Decimal String(number=w701) -> (decimal integer string=w699:string)  [unwired: 1 in]
                        n235 = Number To Decimal String(number=w702) -> (decimal integer string=w687:string)  [unwired: 1 in]
                        n236 = call <vilib>:"Space Constant.vi"() -> ("String"=w700:string)
                        n237 = Open/Create/Replace File(file path (use dialog)="Data File Path", operation (0:open)=T5."replace or create") -> (refnum out=w706:refnum<file>)  [unwired: 4 in, 2 out]
                        n238 = Concatenate Strings(w686, "Data was taken on ", w697, w686, "Integration Time is ", w698, w700, "s", w686, "Monochromator gratng # ", w699, "; ", "blazed for ", w687, w700, "nm", w686, w686, w686, w685) -> (w681:string)
                        n239 = Write to Text File(file (use dialog)=w706, text=w681) -> (refnum out=w671:refnum<file>)  [unwired: 2 in, 2 out]
                        n240 = Flush File(refnum=w671) -> (refnum out=w670:refnum<file>)  [unwired: 1 in, 1 out]
                        n241 = Close File(refnum=w670) -> ()  [unwired: 1 in, 2 out]
                      }
                    }
                    n242 = Build Array (concatenate)(w557, w555) -> (w556:dbl[])
                    n243 = Bundle(w559, w556) -> (w554:cluster{dbl[], dbl[]})  [unwired: 1 in]
                    "Spectrum" <- w554
                    n244 = Unbundle(w554) -> (w553:dbl[], w558:dbl[])
                  }
                }
                frame #1 {
                  n245 = Array Size(array="Array") -> (size(s)=w714:i32)
                  n246 = flat-sequence {
                    tunnel: w712 -> [w721]
                    tunnel: "Array" -> [w720]
                    tunnel: w714 -> [w719]
                    tunnel: [w717] -> w715
                    frame #0 {
                      n247 = for {
                        N: w719 -> [_]
                        tunnel: w720 -> [w732]
                        tunnel: w721 -> [w727]
                        shift-right: [w722] -> w717
                        shift-left: dbl[] [] -> [w723]
                        i -> [w725]
                        n248 = local read "Scan from"() -> (w730:i32)
                        n249 = Index Array(array=w732, index=w725) -> (element=w731:dbl)
                        n250 = local read "Step size"() -> (w728:dbl)
                        n251 = Subtract(x=w731, y=w730) -> (x-y=w729:dbl)
                        n252 = Divide(x=w729, y=w728) -> (x/y=w726:dbl)
                        n253 = Index Array(array=w727, index=w726) -> (element=w724:dbl)
                        n254 = Insert Into Array(array=w723, index=w725, new element=w724) -> (w722:dbl[])
                      }
                    }
                  }
                }
              }
              n255 = local read "Scan from"() -> (w437:i32)
              n256 = local read "Step size"() -> (w435:dbl)
              n257 = To Time Stamp(1:w437) -> (0:w436:timestamp)
              n258 = Bundle By Name("Y"=w441, "t0"=w436, "dt"=w435) -> (w438:waveform(dbl))  [unwired: 1 in]
              n259 = Build Array (concatenate)(w440, w438) -> (w439:waveform(dbl)[])
              "Waveform Graph" <- w439
              n260 = for {
                N: w425 -> [_]
                tunnel: [w481] -> w433
                tunnel: w431 -> [w480]
                tunnel: w428 -> [w478]
                tunnel: [w477] -> w427
                tunnel: w426 -> [w479]
                tunnel: [w474] -> w424 mode=indexing
                i -> [w476]
                n261 = Build Array (concatenate)(w479, w478) -> (w477:dbl[][])
                n262 = Index Array(array=w478, index=w476) -> ()  [unwired: 1 out]
                n263 = Index Array(array=w477, index (col)=w476) -> (element=w475:dbl[])  [unwired: 1 in]
                n264 = Bundle(w480, w475) -> (w474:cluster{dbl[], dbl[]})  [unwired: 1 in]
                n265 = Unbundle(w474) -> (w481:dbl[])  [unwired: 1 out]
              }
              "Decay" <- w424
              "Current Point" <- w421
            }
            n266 = property on="Decay" class="XYGraph (strict)"("XScale.Increment"=w361, "XScale.Maximum"=w391, "XScale.Minimum"=w360) -> ()  [unwired: 2 in, 2 out]
            n267 = Build Array (concatenate)(0, w404) -> ()  [unwired: 1 out]
          }
        }
      }
    }
  }
  n268 = call "Configure.vi"("Dwell Time (s)"="Time between measurements\n at one point (s)/Dwell Time", "Channel T Input"="Trigger mode", "Channel B Input"="Channel B Input", "Channel A Input"="Channel A Input", "Integrating time, 10^-7 sec"="Integrating time \nin 10^-7 sec", "gate mode (CW:0)"="gate mode (CW:0)", "Scan End Mode"=FALSE, "Number of Periods"="Number of Measurements\n to take at one point/ Number of Periods", "Count Mode"="Count Mode", "GPIB Address"="GPIB address") -> ()
  "Mono port" <- w10
  "Time delay" <- w9
